vi "dispose.vi"(8 "error in (no error)":errorcluster, 11 "File Log Provider in":refnum<class "File Log Provider.lvclass">) -> (0 "error out":errorcluster)   [LabVIEW 2019, in "File Log Provider.lvclass"]
uses:
  File Log Provider.lvclass
  File Log Provider.lvclass/File Log Provider.ctl
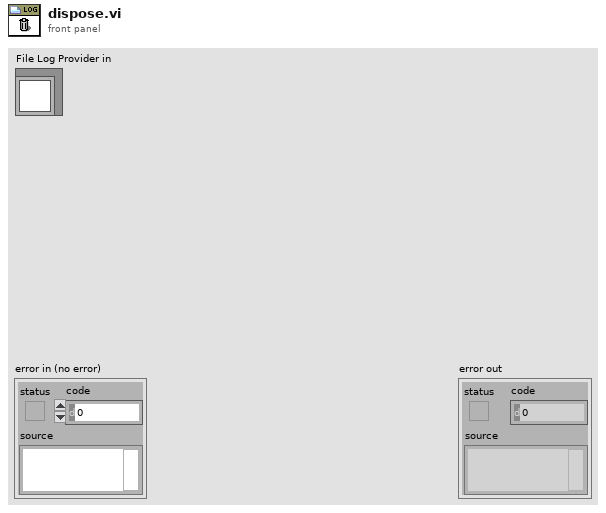
[diagram p1: front panel]
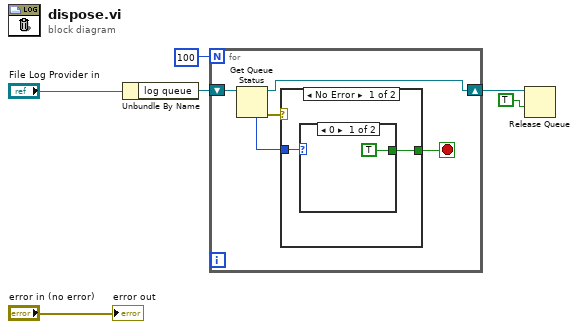
[diagram p0: block diagram]
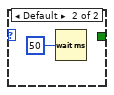
[diagram p2: hidden frame]
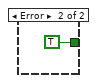
[diagram p3: hidden frame]
diagram:
  n1 = Unbundle By Name("File Log Provider in") -> ("log queue"=w5:refnum<queue>)
  n2 = for {
    N: 100 -> [_]
    shift-right: [w7] -> w2
    shift-left: w5 -> [w11]
    stop <- w9 stop-if-true
    n3 = Get Queue Status(queue=w11) -> (queue out=w7:refnum<queue>, error out=w10:errorcluster, # elements in queue=w8:i32)  [unwired: 2 in, 5 out]
    n4 = case shown="No Error" w10 {
      tunnel: [w12 TRUE] -> w9
      tunnel: w8 -> [w13 _]
      frame No Error {
        n5 = case shown="0" w13 {
          tunnel: [TRUE _] -> w12
          frame 0 {
          }
          frame Default {
            n6 = Wait (ms)(milliseconds to wait=u32 50) -> ()  [unwired: 1 out]
          }
        }
      }
      frame Error {
      }
    }
  }
  n7 = Release Queue(queue=w2, force destroy? (F)=TRUE) -> ()  [unwired: 1 in, 3 out]
  "error out" <- "error in (no error)"
